vi "WriteSignalToTXT.vi"(8 "error in":errorcluster, 10 "waveform":waveform(dbl), 11 "file path in":path) -> (0 "error out":errorcluster, 3 "file path out":path)   [LabVIEW 2025]
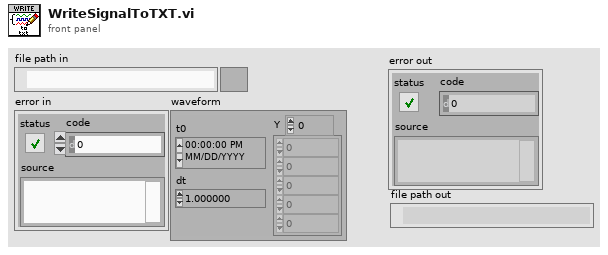
[diagram p1: front panel]
types:
  T1 = enum16{"open", "replace", "create", "open or create", "replace or create", "replace or create with confirmation"}
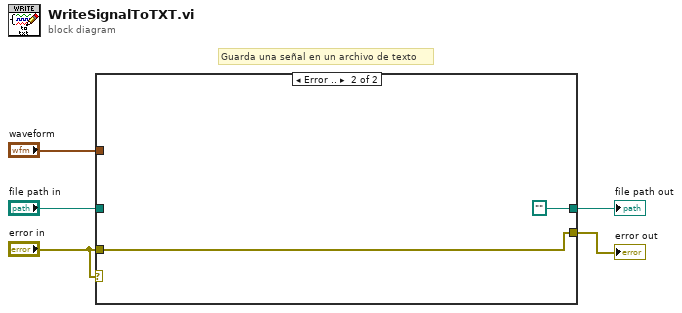
[diagram p0: block diagram]
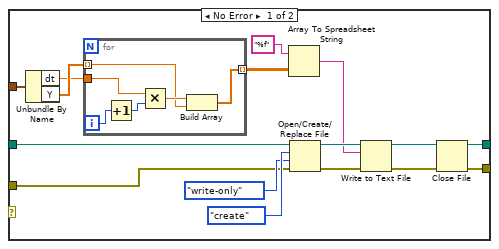
[diagram p2: hidden frame]
diagram:
  # "Guarda una señal en un archivo de texto"
  n1 = case shown="Error .." "error in" {
    tunnel: [w10 w29] -> w5
    tunnel: [w9 path ""] -> w4
    tunnel: "file path in" -> [w8 _]
    tunnel: "error in" -> [w7 w29]
    tunnel: "waveform" -> [w6 _]
    frame No Error {
      n2 = Unbundle By Name(w6) -> ("dt"=w15:dbl, "Y"=w16:dbl[])
      n3 = for {
        tunnel: w16 -> [w22] mode=indexing
        tunnel: w15 -> [w23]
        tunnel: [w24] -> w14 mode=indexing
        i -> [w27]
        n4 = Increment(x=w27) -> (x+1=w26:i32)
        n5 = Multiply(x=w23, y=w26) -> (x*y=w25:dbl)
        n6 = Build Array(w25, w22) -> (w24:dbl[])
      }
      n7 = Array To Spreadsheet String(array=w14, 3:"%f" ("format string")) -> (spreadsheet string=w13:string)  [unwired: 1 in]
      n8 = Open/Create/Replace File(file path (use dialog)=w8, error in=w7, operation (0:open)=T1."create", access (0:read/write)=enum16{"read/write", "read-only", "write-only"}."write-only") -> (refnum out=w19:refnum<file>, error out=w18:errorcluster)  [unwired: 2 in, 1 out]
      n9 = Write to Text File(file (use dialog)=w19, text=w13, error in=w18) -> (refnum out=w12:refnum<file>, error out=w11:errorcluster)  [unwired: 1 in, 1 out]
      n10 = Close File(refnum=w12, error in=w11) -> (path=w9:path, error out=w10:errorcluster)
    }
    frame Error {
    }
  }
  "error out" <- w5
  "file path out" <- w4
